vi "SetupInterf.vi"(8 "error in (no error)":errorcluster caption="entrée d'erreur (pas d'erreur)", 9 "Experiment.lvclass":refnum<class "Experiment.lvclass">=refnum, 11 "Interface en entrée":refnum<class "Interface.lvclass"> caption="Interface Class in") -> (0 "error out":errorcluster caption="sortie d'erreur", 3 "Interface en sortie":refnum<class "Interface.lvclass"> caption="DNL_LabVIEW Object out")   [LabVIEW 2019, in "Interface.lvclass"]
uses:
  Interface.lvclass
  Experiment Class/Experiment.lvclass
  DevicesClass/Tools/Tools.lvclass
  CurveSetup.ctl
  SetupInterfStates.ctl
  Interface.lvclass/Interface.ctl
  SetInitPar.ctl
  2DGraphSetup.ctl
  DevicesClass/BaseDevice/BaseDevice.lvclass
panel:
  out "ScanInstrInd":i32[][](array[numeric])
  out "ArrDev":bool[](array[boolean])
  in  "EditArrDev":bool
  out "2D Scan":bool
  in  "2D Plot Act":bool caption="2D Plot"
  out "Fill Line First":bool
  in  "2D Plot":bool
  in  "2D YScanPar":u16(ring) caption="Y Parameter" items=["Selectionner un Paramètre..", "Tools.ScanPar(Arb)"]
  in  "2D XScanPar":u16(ring) caption="X Parameter" items=["Selectionner un Paramètre..", "Tools.Ind Point(Point)", "Tools.ScanPar(Arb)"]
  in  "Data Only":bool
  in  "SaveNamingPar":bool
  out "GraphIndex":i32
  in  "SetGraphConf":bool
  out "Graph Config":i32
  in  "2ndVarParPos":bool=TRUE caption="2nd Scan Parameter Position"
  in  "2ndScanParName":bool=TRUE caption="2nd Scan Parameter Name"
  in  "ParamNaming":bool caption="Use Parameterize Naming"
  in  "YScale":u32(ring) items=["Left 1", "Left 2", "Left 3", "Right 1", "Right 2", "Right 3"]
  in  "X Scale":u32(ring) items=["Bottom", "Top"]
  in  "ScanInstrName":bool=TRUE
  in  "Scan/Log Suffix":bool=TRUE
  in  "MeasUnits":bool=TRUE caption="Measurement Units"
  in  "MeasInstrName":bool=TRUE
  in  "SaveCurvePar":bool
  in  "DisplayName":string
  in  "Visible":bool
  out "CrvParOut":T1[](array[typedef])
  out "NomDon":string[](array[string])=["RTêta;", "X&Y;"]
  out "VarParams":string[][](array[string])
  in  "AutoColor":bool caption="Use Automatic Color"
  out "Graphe XY":cluster{dbl, dbl}[](graph)
  in  "ScanParam":u16(ring) caption="Scan Parameter" items=["Tools.Ind Point(Point)"]
  in  "YScaleName":string
  in  "XScaleName":string
  in  "Graph Window":i32(ring) items=["Graph 0", "No Graph", "New Graph Window "]
  in  "stop":bool
  in  "Curve List":i32(listbox)
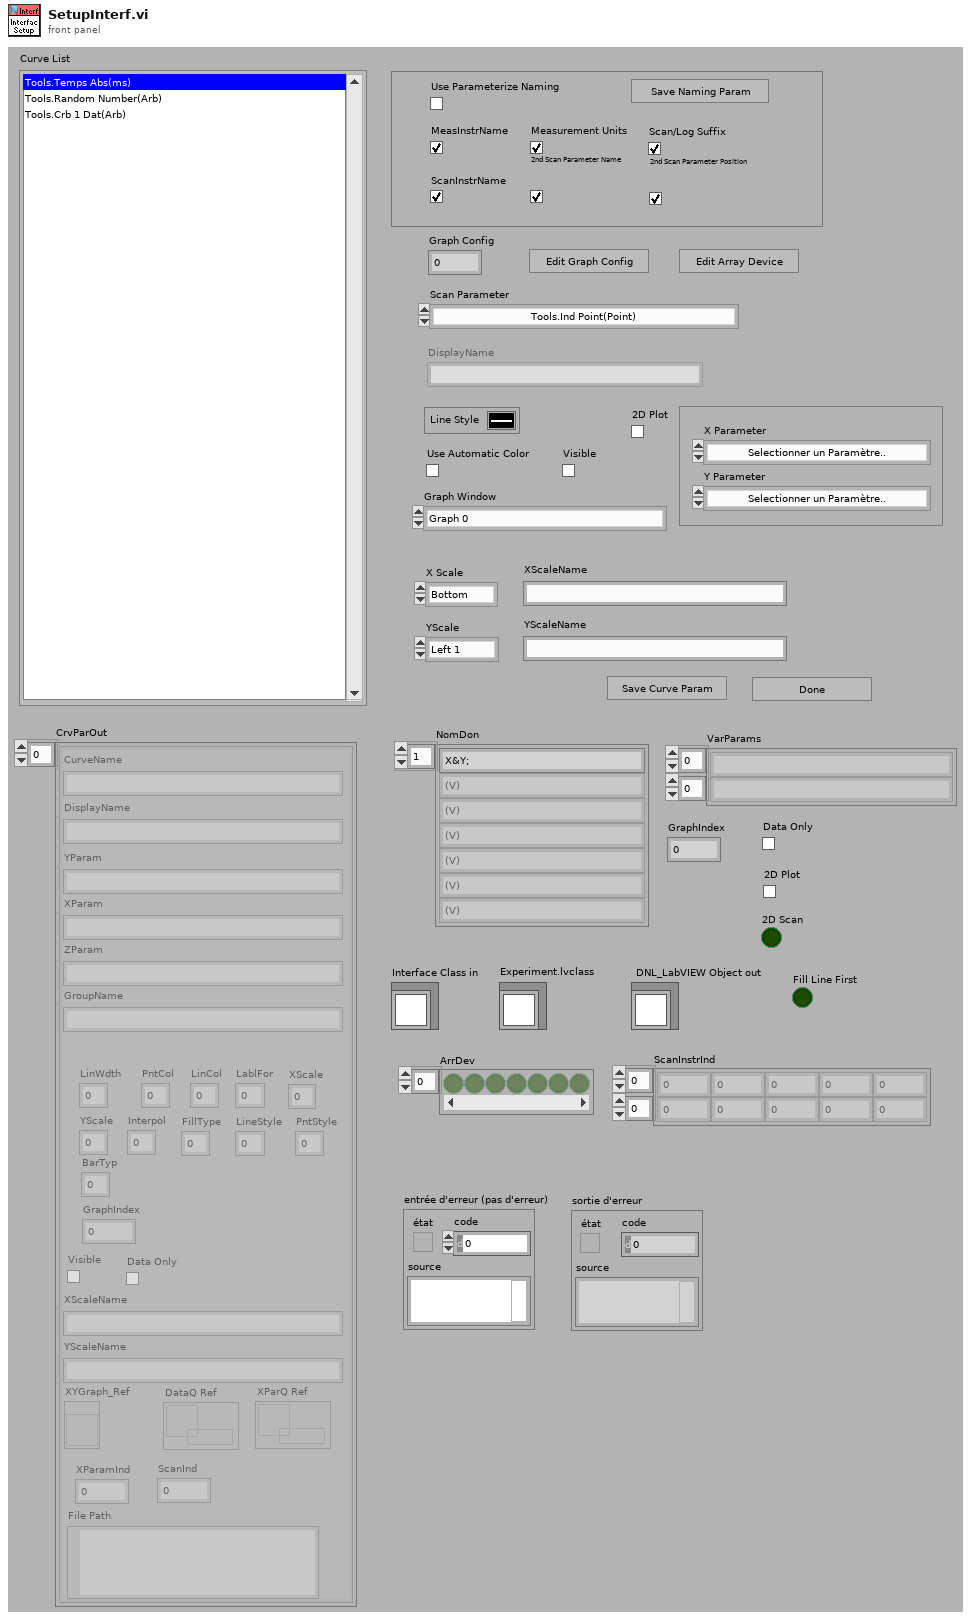
[diagram p1: front panel]
types:
  T1 = typedef "Interface.lvclass/CurveSetup.ctl" = cluster{"CurveName":string, "YParam":string, "XParam":string, "ZParam ":string, "GroupName":string, "LinWdth":u8, "PntCol":u32, "LinCol":u32, "LablFor":u8, "XScale":u32, "YScale":u32, "Interpol":u8, "DisplayName":string, "FillType":i16, "LineStyle":u8, "PntStyle":u8, "BarTyp":u8, "GraphIndex":i32, "Visible":bool, "XScaleName":string, "YScaleName":string, "XYGraph_Ref":refnum<vi>, "Data Only":bool, "DataQ Ref":refnum<queue>, "XParQ Ref":refnum<queue>, "XParamInd":i32, "ScanInd":i32, "File Path":path}
  T2 = typedef "SetInitPar.ctl" = enum16{"All", "AllowSave", "GraphConfig", "ScanFormats", "ScanPref", "LogPref", "BasePath", "Experiment", "SubFolder"}
  T3 = cluster{"MeasInstrNm":bool, "MeasUnits":bool, "ScanSuff":bool, "ScanParNm":bool, "2ndScnParNm":bool, "2ndScnParPos":bool}
  T4 = typedef "SetupInterfStates.ctl" = enum16{"InitProg", "ReadMeasPar", "ReadCurvePar", "ReadGraphPar", "GetScaleName", "ChgScaleName", "ChngGraphConf", "2D Graph", "SaveParams", "SaveParamsDef", "ApplyAll", "ArrDevSetup", "Stop"}
  T5 = enum16{"Enable", "Disable", "DisAndGrayed", "ReinitToDefVal"}
  T6 = enum16{"Enable", "Disable", "DisAndGrayed", "ReinitToDefVal", "EnumElementsArr"}
  T7 = typedef "2DGraphSetup.ctl" = cluster{"ZDataIndex":i32, "XParIndex":i32, "YParIndex":i32, "FillLineFirst":bool, "2DGraphIndex":i32, "XParQ Ref":refnum<queue>, "YParQ Ref":refnum<queue>, "DataQRefs":refnum<queue>[], "CurveName":string, "XparInstrInd":i32, "YparInstrInd":i32, "Active":bool}
  T8 = enum32{"Invalid", "Standard", "Closed", "Hidden", "Minimized", "Maximized"}
  T9 = enum8{"Enabled", "Disabled", "Disabled and Grayed Out"}
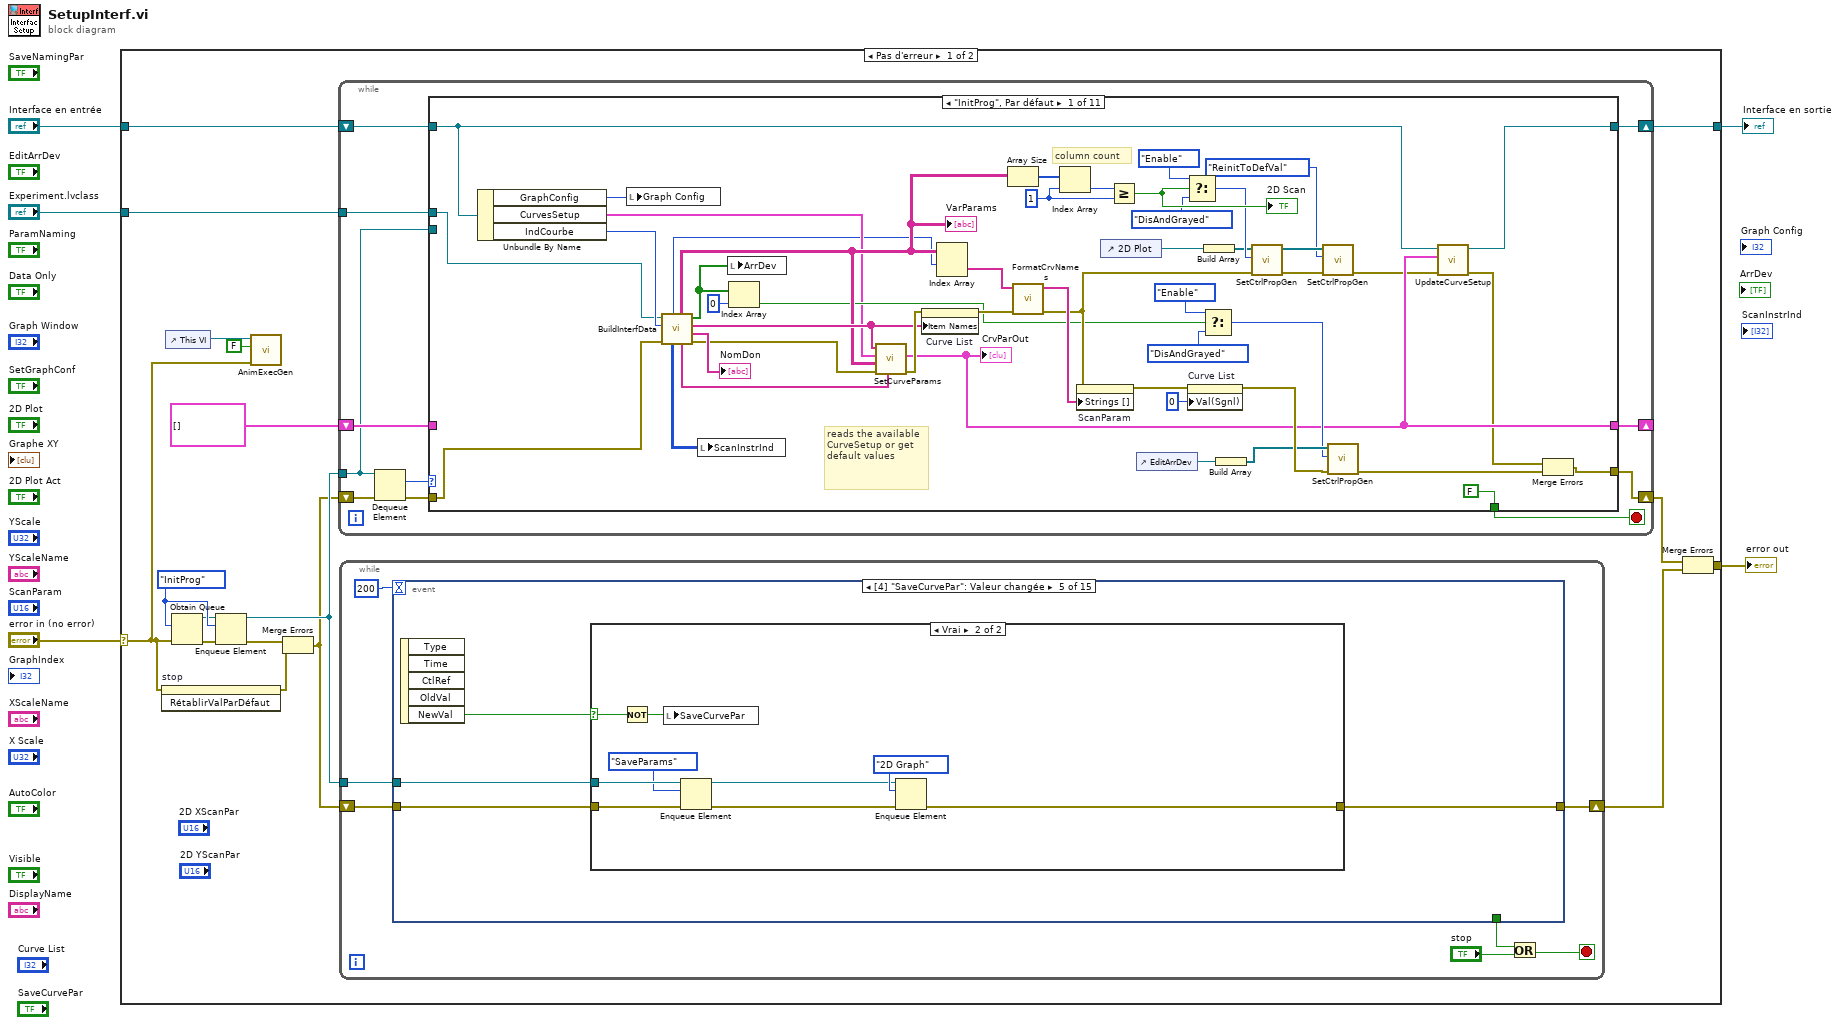
[diagram p0: block diagram]
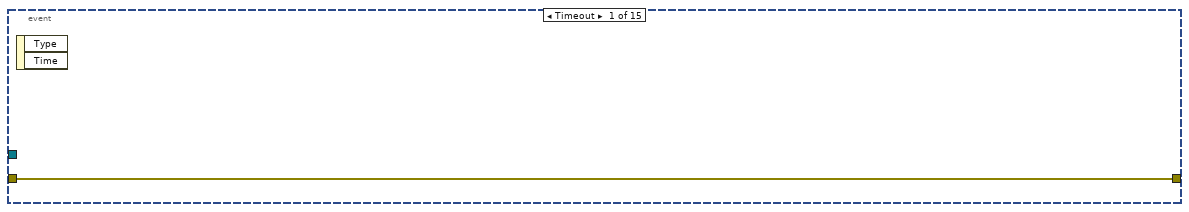
[diagram p2: hidden frame]
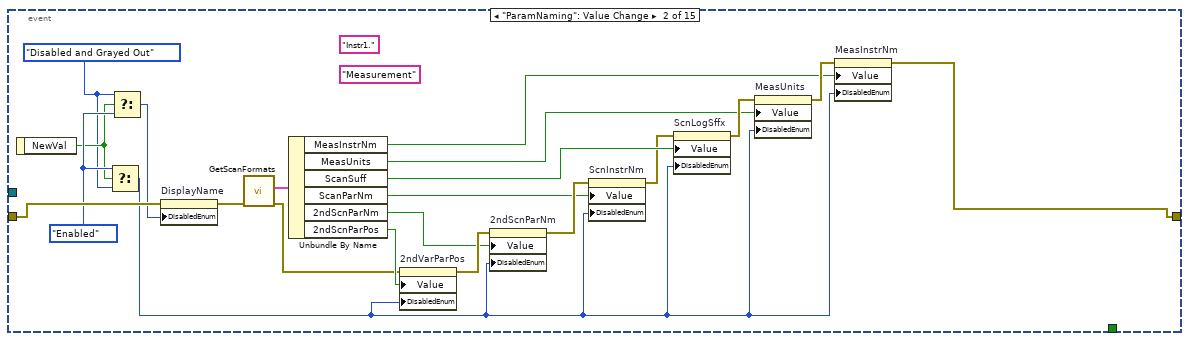
[diagram p3: hidden frame]
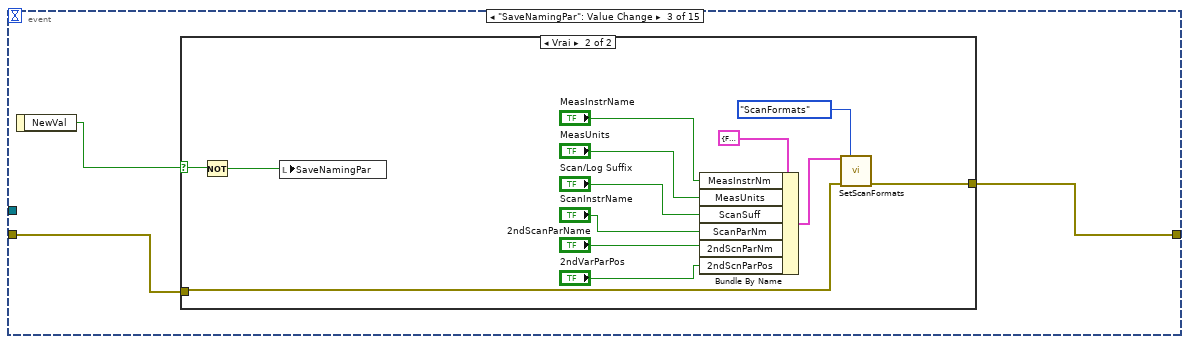
[diagram p4: hidden frame]
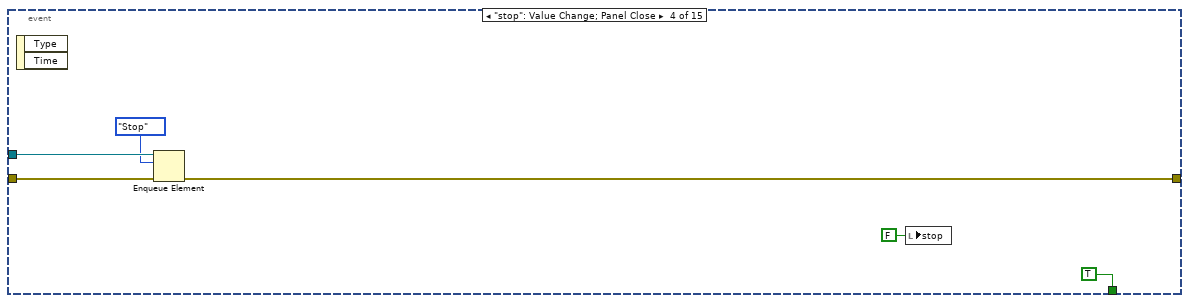
[diagram p6: hidden frame]
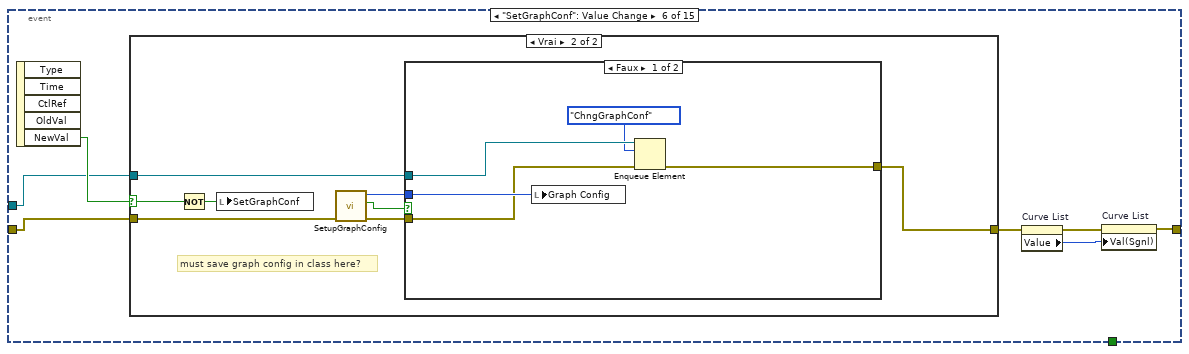
[diagram p8: hidden frame]
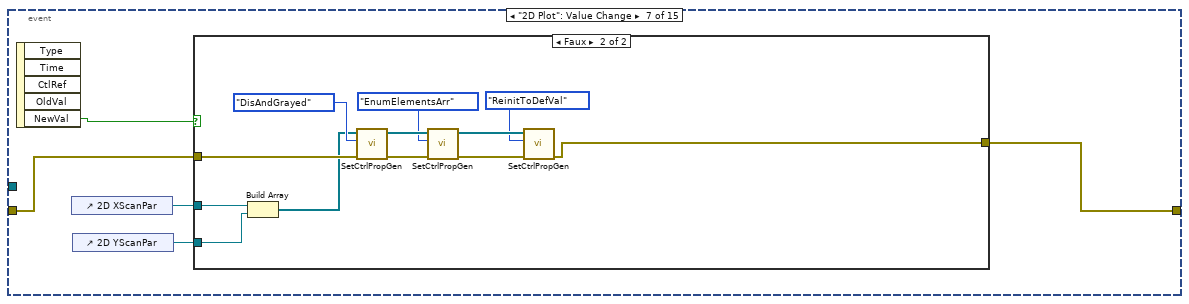
[diagram p11: hidden frame]
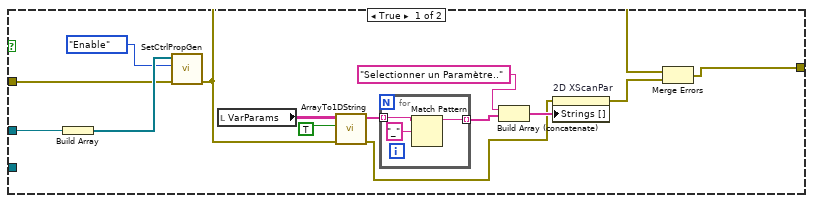
[diagram p12: hidden frame]
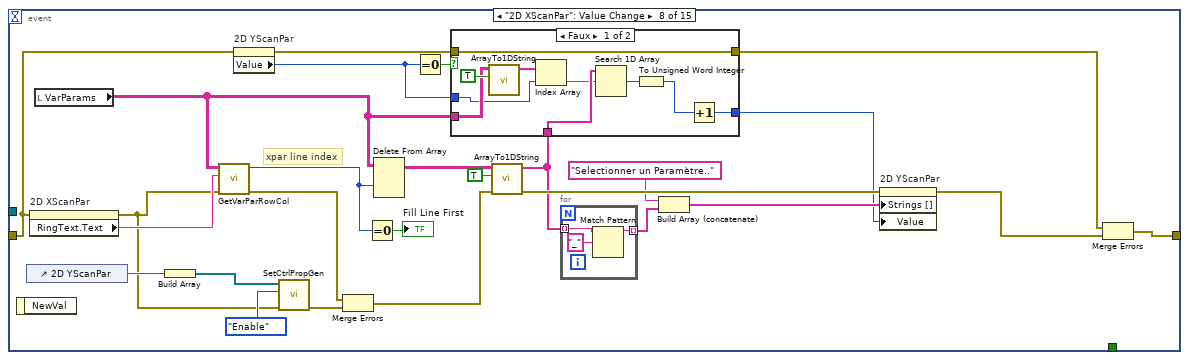
[diagram p13: hidden frame]
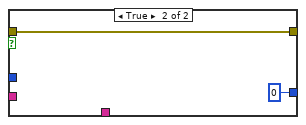
[diagram p14: hidden frame]
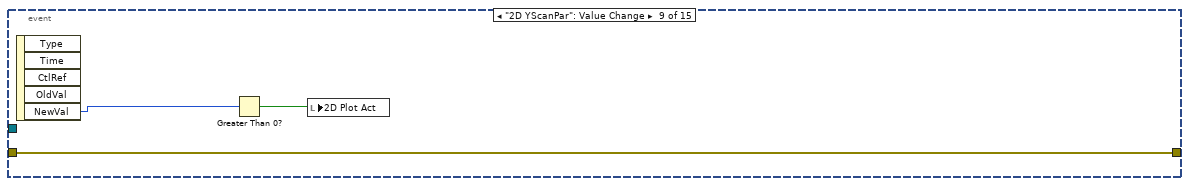
[diagram p15: hidden frame]
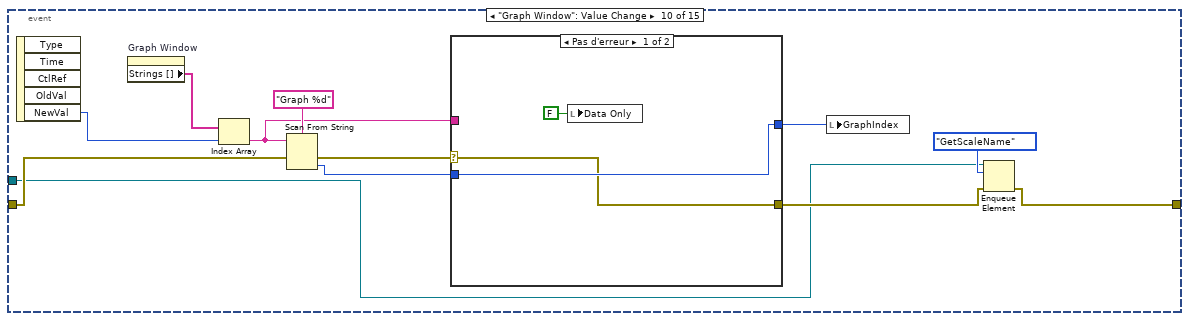
[diagram p16: hidden frame]
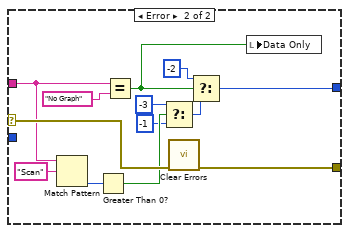
[diagram p17: hidden frame]
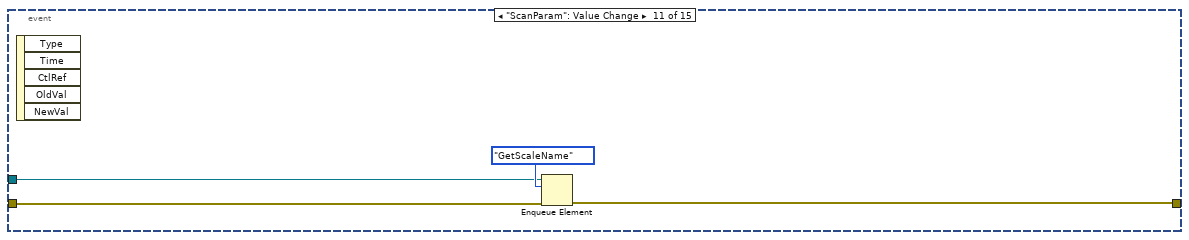
[diagram p18: hidden frame]
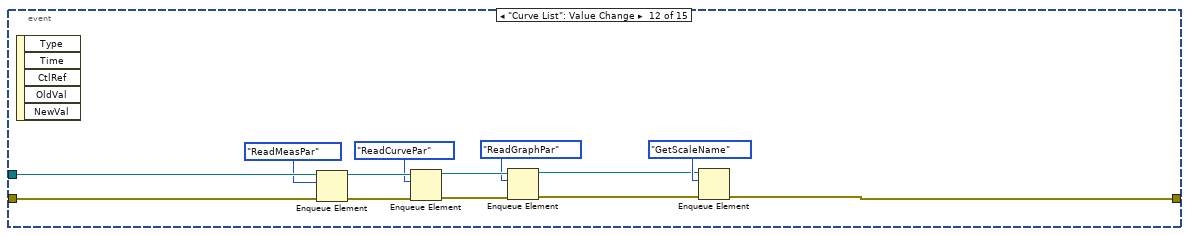
[diagram p19: hidden frame]
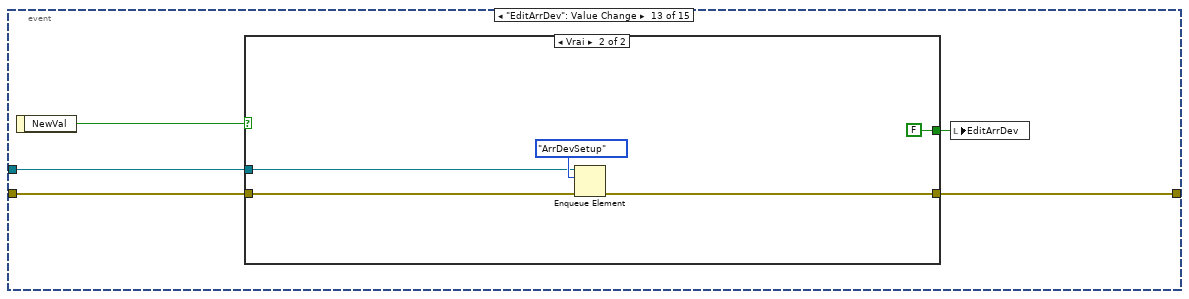
[diagram p20: hidden frame]
diagram:
  n1 = case shown="Pas d'erreur" "error in (no error)" {
    selector: "error in (no error)" -> [w7 w726]
    tunnel: [w11 w726] -> w4
    tunnel: "Interface en entrée" -> [w14 w725]
    tunnel: [w6 w725] -> w2
    tunnel: "Experiment.lvclass" -> [w10 _]
    frame No Error {
      w22 = SetupInterfStates."InitProg" ("Énum")
      n2 = invoke on="stop" class="Bool (strict)" method="RétablirValParDéfaut"(error in=w7) -> (error out=w16:errorcluster)  [unwired: 2 in, 2 out]
      n3 = control-ref of="This VI"() -> (w8:refnum<vi>)
      n4 = Obtain Queue(element data type=w22, error in (no error)=w7) -> (queue out=w21:refnum<queue>, error out=w20:errorcluster)  [unwired: 3 in, 1 out]
      n5 = Enqueue Element(queue=w21, element=w22, error in (no error)=w20) -> (queue out=w19:refnum<queue>, error out=w17:errorcluster)  [unwired: 1 in, 1 out]
      n6 = call <userlib>:"AnimExecGen.vi"("ErrorIn(No Error)"=w7, "Animer l'exécution ?"=FALSE, "ViRef"=w8) -> ()  [unwired: 8 in, 1 out]
      n7 = Merge Errors(w17, w16) -> (w15:errorcluster)
      n8 = while {
        shift-right: [w258] -> w12
        shift-left: w15 -> [w263]
        tunnel: w19 -> [w255]
        shift-right: [w259] -> w6
        shift-left: w14 -> [w262]
        shift-right: [w257] -> _
        shift-left: T1[] [] ("CurveParamsOut") -> [w256]
        tunnel: w10 -> [w254]
        stop <- w260 stop-if-true
        n9 = Dequeue Element(queue=w255, error in (no error)=w263) -> (element=w264:T4, error out=w261:errorcluster)  [unwired: 1 in, 2 out]
        n10 = case shown="\"InitProg\", Par défaut" w264 {
          tunnel: w262 -> [w272 w338 w342 w406 w481 w512 w528 w570 w613 w678 w704]
          tunnel: w261 -> [w267 w332 w365 w425 w492 w519 w530 w567 w631 w672 w693]
          tunnel: [FALSE _ _ _ _ _ _ _ _ TRUE FALSE] -> w260
          tunnel: [w271 w338 w342 w406 w481 w508 w524 w561 w625 w678 w703] -> w259
          tunnel: [w289 w330 w350 w409 w493 w506 w525 w568 w604 w676 w705] -> w258
          tunnel: [w270 w329 w363 w422 w503 w522 w523 w569 w601 w677 w686] -> w257
          tunnel: w256 -> [_ w329 w363 w422 w503 w522 w523 w569 w647 w677 w687]
          tunnel: w255 -> [_ _ _ _ _ _ _ _ _ _ _]
          tunnel: w254 -> [w285 _ _ _ _ _ _ _ _ _ w698]
          frame "InitProg", Default {
            w296 = 1 ("indice")
            # "column count"
            # "reads the available CurveSetup or get default values"
            n11 = Unbundle By Name(w272) -> ("GraphConfig"=w302:i32, "CurvesSetup"=w273:T1[], "IndCourbe"=w301:i64)
            n12 = local write "Graph Config"(w302) -> ()
            n13 = call "BuildInterfData.vi"("error in"=w267, "IndCourbe"=w301, "Experiment.lvclass In"=w285) -> ("error out"=w304:errorcluster, "NomDon"=→"NomDon":string[], "Scan list"=w303:string[], "ArrDev"=w275:bool[], "VarPar list"=w274:string[], "VarParams"=w300:string[][], "ScanInstIndexOut"=w266:i32[][], "firstenableSProw"=w265:i32)  [unwired: 1 in]
            "VarParams" <- w300
            n14 = local write "ScanInstrInd"(w266) -> ()
            n15 = local write "ArrDev"(w275) -> ()
            n16 = Index Array(array=w275, index=0 ("indice")) -> (element=w279:bool)
            n17 = call "SetCurveParams.vi"("VarPar list"=w274, "error in (no error)"=w304, "VarParams"=w300, "CurveSetupsIn"=w273, "CurveNames"=w303) -> ("error out"=w311:errorcluster, "CurveSetupsOut"=w270:T1[])  [unwired: 5 in]
            "CrvParOut" <- w270
            n18 = property on="Curve List" class="LstDér (strict)"(error in=w311, "Item Names"=w303) -> (error out=w305:errorcluster)  [unwired: 1 in, 1 out]
            n19 = Index Array(array=w300, index (row)=w265) -> (element=w307:string[])  [unwired: 1 in]
            n20 = Array Size(array=w300) -> (size(s)=w299:i32[])
            n21 = call "FormatCrvNames.vi"("entrée d'erreur"=w305, "CurveNamesIn"=w307) -> ("sortie d'erreur"=w290:errorcluster, "CurveNames"=w306:string[])  [unwired: 8 in]
            n22 = Index Array(array=w299, index=w296) -> (element=w297:i32)
            n23 = property on="ScanParam" class="MDér (strict)"(error in=w290, "Strings []"=w306) -> (error out=w308:errorcluster)  [unwired: 1 in, 1 out]
            n24 = control-ref of="2D Plot"() -> (w291:refnum<vi>)
            n25 = Greater Or Equal?(x=w297, y=w296) -> (x >= y?=w298:bool)
            "2D Scan" <- w298
            n26 = control-ref of="EditArrDev"() -> (w281:refnum<vi>)
            n27 = Select(t=T5."Enable" ("Énum"), s=w298, f=T5."DisAndGrayed" ("Énum")) -> (s? t:f=w294:T5)
            n28 = property on="Curve List" class="LstDér (strict)"(error in=w308, "Val(Sgnl)"=0 ("Valeur (Signalisation)")) -> (error out=w283:errorcluster)  [unwired: 1 in, 1 out]
            n29 = Select(t=T5."Enable" ("Énum"), s=w279, f=T5."DisAndGrayed" ("Énum")) -> (s? t:f=w276:T5)
            n30 = Build Array(w291) -> (w293:refnum<vi>[])
            n31 = Build Array(w281) -> (w280:refnum<vi>[])
            n32 = call <userlib>:"SetCtrlPropGen.vi"("Error in"=w290, "Énum"=w294, "Controls"=w293) -> ("Error out"=w286:errorcluster, "Controls Out"=w288:refnum<vi>[])  [unwired: 3 in]
            n33 = call <userlib>:"SetCtrlPropGen.vi"("Error in"=w286, "Énum"=T5."ReinitToDefVal", "Controls"=w288) -> ("Error out"=w269:errorcluster)  [unwired: 3 in, 1 out]
            n34 = call <userlib>:"SetCtrlPropGen.vi"("Error in"=w283, "Énum"=w276, "Controls"=w280) -> ("Error out"=w282:errorcluster)  [unwired: 3 in, 1 out]
            n35 = call "UpdateCurveSetup.vi"("ErrorIn(No Error)"=w269, "CurveSetupsIn"=w270, "Interface.lvclass"=w272) -> ("sortie d'erreur"=w268:errorcluster, "Interface.lvclass Out"=w271:refnum<class "Interface.lvclass">)  [unwired: 7 in]
            n36 = Merge Errors(w268, w282) -> (w289:errorcluster)
          }
          frame "ReadMeasPar" {
            n37 = property on="Curve List" class="LstDér (strict)"(error in=w332) -> (error out=w314:errorcluster, "Value"=w316:i32)  [unwired: 1 in, 1 out]
            n38 = local read "ArrDev"() -> (w317:bool[])
            n39 = control-ref of="EditArrDev"() -> (w321:refnum<vi>)
            n40 = Index Array(array=w317, index=w316) -> (element=w315:bool)
            n41 = Build Array(w321) -> (w320:refnum<vi>[])
            n42 = Select(t=T5."Enable" ("Énum"), s=w315, f=T5."DisAndGrayed" ("Énum")) -> (s? t:f=w322:T5)
            n43 = call <userlib>:"SetCtrlPropGen.vi"("Error in"=w314, "Énum"=w322, "Controls"=w320) -> ("Error out"=w313:errorcluster)  [unwired: 3 in, 1 out]
            n44 = Index Array(array=w329, index=w316) -> (element=w331:T1)
            n45 = property on="ScanParam" class="MDér (strict)"(error in=w313) -> (error out=w324:errorcluster, "Strings []"=w333:string[])  [unwired: 1 in, 1 out]
            n46 = Unbundle By Name(w331) -> ("XParam"=w328:string)  [unwired: 1 out]
            n47 = Build Array(w328) -> (w327:string[])
            n48 = call "FormatCrvNames.vi"("entrée d'erreur"=w324, "CurveNamesIn"=w327) -> ("sortie d'erreur"=w323:errorcluster, "CurveNames"=w326:string[])  [unwired: 8 in]
            n49 = Index Array(array=w326) -> (element=w325:string)  [unwired: 1 in]
            n50 = Search 1D Array(1D array=w333, element=w325) -> (index of element=w336:i32)  [unwired: 1 in]
            n51 = Greater Or Equal To 0?(x=w336) -> (x >= 0?=w334:bool)
            n52 = Select(t=w336, s=w334, f=0 ("cas faux")) -> (s? t:f=w337:i32)
            n53 = property on="ScanParam" class="MDér (strict)"(error in=w323, "Value"=w337) -> (error out=w330:errorcluster)  [unwired: 1 in, 1 out]
          }
          frame "ReadCurvePar" {
            n54 = Unbundle By Name(w342) -> ("2DGphParams"=w343:T7[])
            n55 = property on="Curve List" class="LstDér (strict)"(error in=w365) -> (error out=w353:errorcluster, "Item Names"=w347:string[], "Value"=w345:i32)  [unwired: 1 in, 1 out]
            n56 = Index Array(array=w347, index=w345) -> (element=w346:string)
            n57 = Index Array(array=w363, index=w345) -> (element=w366:T1)
            n58 = for {
              tunnel: w343 -> [w380] mode=indexing
              tunnel: w346 -> [w378]
              tunnel: [w377] -> w344
              tunnel: [w376] -> w341
              tunnel: [w375] -> w340
              i -> [w377]
              stop <- w376 stop-if-true
              n59 = Unbundle By Name(w380) -> ("Active"=w375:bool, "CurveName"=w379:string)
              n60 = Equal?(x=w379, y=w378) -> (x = y?=w376:bool)
            }
            n61 = Unbundle By Name(w366) -> ("PntCol"=w362:u32, "LinCol"=w361:u32)
            n62 = And(x=w340, y=w341) -> (x .and. y?=w339:bool)
            n63 = Unbundle By Name(w366) -> ("LinWdth"=w374:u8, "LablFor"=w368:u8)
            n64 = Unbundle By Name(w366) -> ("Interpol"=w369:u8, "FillType"=w370:i16, "LineStyle"=w371:u8, "PntStyle"=w372:u8, "BarTyp"=w373:u8)
            n65 = call "GetPlotColors.vi"("Color2In"=w361, "Color1In"=w362, "ColorIndex"=0) -> ("Color2Out"=w357:u32, "Color1Out"=w358:u32, "AutoColor"=w359:bool)  [unwired: 5 in, 1 out]
            n66 = local write "AutoColor"(w359) -> ()
            n67 = Index Array(array=w343, index=w344) -> (element=w348:T7)
            n68 = property on="Graphe XY" class="GraphXY (strict)"(error in=w353, "Active Plot"=u32 0 ("Tracé actif"), "Plot.Fill/Pt. Color"=w358, "Plot.Plot Color"=w357, "Plot.Line Width"=w374, "Plot.Label Style"=w368, "Plot.Plot Interpolation"=w369, "Plot.Fill To"=w370, "Plot.Line Style"=w371, "Plot.Point Style"=w372, "Plot.Bar Plot Style"=w373) -> (error out=w364:errorcluster)  [unwired: 1 in, 1 out]
            n69 = Unbundle By Name(w348) -> ("ZDataIndex"=w354:i32, "XParIndex"=w352:i32, "YParIndex"=w351:i32)
            n70 = call <vilib>:"General Error Handler.vi"("error in (no error)"=w364) -> ("error out"=w356:errorcluster)  [unwired: 10 in, 4 out]
            n71 = case shown="Vrai" w339 {
              tunnel: w354 -> [_ _]
              tunnel: w353 -> [w382 w389]
              tunnel: w352 -> [_ w392]
              tunnel: w351 -> [_ w385]
              tunnel: [w381 w387] -> w349
              frame False {
                n72 = property on="2D Plot" class="Bool (strict)"(error in=w382, "Val(Sgnl)"=FALSE ("Valeur (Signalisation)")) -> (error out=w381:errorcluster)  [unwired: 1 in, 1 out]
              }
              frame True {
                n73 = property on="2D Plot" class="Bool (strict)"(error in=w389, "Val(Sgnl)"=TRUE ("Valeur (Signalisation)")) -> (error out=w393:errorcluster)  [unwired: 1 in, 1 out]
                n74 = Increment(x=w392) -> (x+1=w391:i32)
                n75 = To Unsigned Word Integer(number=w391) -> (unsigned 16bit integer=w390:u16)
                n76 = property on="2D XScanPar" class="MDér (strict)"(error in=w393, "Val(Sgnl)"=w390) -> (error out=w388:errorcluster)  [unwired: 1 in, 1 out]
                n77 = To Unsigned Word Integer(number=w385) -> (unsigned 16bit integer=w384:u16)
                n78 = property on="2D YScanPar" class="MDér (strict)"(error in=w388, "Value"=w384) -> (error out=w387:errorcluster)  [unwired: 1 in, 1 out]
              }
            }
            n79 = local write "2D Plot Act"(w339) -> ()
            n80 = call <vilib>:"Clear Errors.vi"("error in (no error)"=w356) -> ("error out"=w355:errorcluster)  [unwired: 5 in, 1 out]
            n81 = Merge Errors(w349, w355) -> (w350:errorcluster)
          }
          frame "ReadGraphPar" {
            n82 = local read "Graph Config"() -> (w399:i32)
            n83 = property on="Curve List" class="LstDér (strict)"(error in=w425) -> (error out=w416:errorcluster, "Value"=w405:i32)  [unwired: 1 in, 1 out]
            n84 = Index Array(array=w422, index=w405) -> (element=w423:T1)
            n85 = local read "2D Scan"() -> (w395:bool)
            n86 = Unbundle By Name(w423) -> ("GraphIndex"=w417:i32)
            n87 = call "GraphConfCount.vi"("Configuration"=w399) -> ("GraphCount"=w398:i32)  [unwired: 9 in, 1 out]
            n88 = To Long Integer(number=w398) -> (32bit integer=w418:i32)
            n89 = Greater Or Equal To 0?(x=w417) -> (x >= 0?=w419:bool)
            n90 = Select(t=string[] ["No Graph", "New Graph Window For Each Curve", "New Graph Window For Each Scan"], s=w395, f=string[] ["No Graph", "New Graph Window "]) -> (s? t:f=w397:string[])
            n91 = case shown="Vrai" w419 {
              tunnel: w418 -> [w428 w455]
              tunnel: w417 -> [w426 w457]
              tunnel: [w433 w460] -> w415
              tunnel: w416 -> [w432 w459]
              tunnel: [w430 w458] -> w414
              tunnel: w397 -> [w429 w454]
              tunnel: [w431 w456] -> w413
              tunnel: [w427 w453] -> w412
              frame False {
                # "either new window (-1,-3) or no window(-2)"
                n92 = Equal?(x=w426, y=-2) -> (x = y?=w434:bool)
                n93 = case shown="Faux" w434 {
                  tunnel: [w446 w452] -> w433
                  tunnel: w432 -> [w446 w452]
                  tunnel: w428 -> [w445 w451]
                  tunnel: [w448 w451] -> w431
                  tunnel: [w447 w450] -> w430
                  tunnel: w429 -> [w447 w450]
                  tunnel: [w438 -2] -> w427
                  tunnel: w426 -> [w444 _]
                  frame False {
                    n94 = Equal?(x=w444, y=-1) -> (x = y?=w439:bool)
                    n95 = Select(t=1 ("y"), s=w439, f=2 ("y")) -> (s? t:f=w440:i32)
                    n96 = Select(t=-1, s=w439, f=-3) -> (s? t:f=w438:i32)
                    n97 = Add(x=w445, y=w440) -> (x+y=w448:i32)
                  }
                  frame True {
                    # "No graph"
                  }
                }
              }
              frame True {
                # "either valid or invalid (absent) graph window"
                n98 = Less Or Equal?(x=w455, y=w457) -> (x <= y?=w461:bool)
                n99 = case shown="Vrai" w461 {
                  tunnel: w459 -> [w464 w473]
                  tunnel: [w464 w472] -> w460
                  tunnel: [w463 w470] -> w458
                  tunnel: w454 -> [w463 w469]
                  tunnel: w457 -> [w462 w465]
                  tunnel: [w462 w466] -> w456
                  tunnel: w455 -> [_ w468]
                  tunnel: [w462 w465] -> w453
                  frame False {
                  }
                  frame True {
                    n100 = Add(x=w468, y=2) -> (x+y=w466:i32)
                    n101 = Format Into String(format string="Graph %d (unavailable)" ("chaîne de format"), error in=w473, w465) -> (resulting string=w471:string, error out=w472:errorcluster)  [unwired: 1 in]
                    n102 = Build Array (concatenate)(w469, w471) -> (w470:string[])
                  }
                }
              }
            }
            n103 = for {
              N: w418 -> [_]
              tunnel: [w475] -> w421 mode=indexing
              i -> [w477]
              n104 = Format Into String(format string="Graph %d" ("chaîne de format"), w477) -> (resulting string=w475:string)  [unwired: 2 in, 1 out]
            }
            n105 = local write "GraphIndex"(w412) -> ()
            n106 = Unbundle By Name(w423) -> ("Data Only"=w408:bool, "DisplayName"=w411:string, "Visible"=w424:bool, "XScale"=w402:u32, "YScale"=w401:u32)
            n107 = Build Array (concatenate)(w421, w414) -> (w420:string[])
            n108 = property on="Graph Window" class="MDér (strict)"(error in=w415, "Strings []"=w420, "Value"=w413) -> (error out=w400:errorcluster)  [unwired: 1 in, 1 out]
            n109 = Empty String/Path?(string/path=w411) -> (empty?=w410:bool)
            n110 = local write "Data Only"(w408) -> ()
            n111 = local write "DisplayName"(w411) -> ()
            n112 = local write "Visible"(w424) -> ()
            n113 = property on="X Scale" class="MDér (strict)"(error in=w400, "Value"=w402) -> (error out=w404:errorcluster)  [unwired: 1 in, 1 out]
            n114 = property on="YScale" class="MDér (strict)"(error in=w400, "Value"=w401) -> (error out=w403:errorcluster)  [unwired: 1 in, 1 out]
            n115 = Merge Errors(w404, w403) -> (w407:errorcluster)
            n116 = property on="ParamNaming" class="Bool (strict)"(error in=w407, "Val(Sgnl)"=w410) -> (error out=w409:errorcluster)  [unwired: 1 in, 1 out]
          }
          frame "GetScaleName" {
            # "if you don't \"save param\"\ngraph stays with no scale"
            # "The first data element gives is names to the y scale #0\nThe first varpar gives is name to the x scale #0\nOther scale number get their names attributed at selection"
            n117 = property on="GraphIndex" class="NumNb (strict)"(error in=w492) -> ("Value"=w487:i32)  [unwired: 1 in, 2 out]
            n118 = property on="Curve List" class="LstDér (strict)"(error in=w492) -> (error out=w479:errorcluster, "Value"=w504:i32)  [unwired: 1 in, 1 out]
            n119 = Index Array(array=w503, index=w504) -> (element=w499:T1)
            n120 = property on="ScanParam" class="MDér (strict)"(error in=w479) -> (error out=w478:errorcluster, "RingText.Text"=w480:string)  [unwired: 1 in, 1 out]
            n121 = Unbundle By Name(w499) -> ("CurveName"=w496:string)
            n122 = property on="X Scale" class="MDér (strict)"(error in=w479) -> (error out=w495:errorcluster, "Value"=w490:u32)  [unwired: 1 in, 1 out]
            n123 = property on="YScale" class="MDér (strict)"(error in=w479) -> (error out=w494:errorcluster, "Value"=w485:u32)  [unwired: 1 in, 1 out]
            n124 = Unbundle By Name(w481) -> ("XScalesNames"=w491:string[][], "YScalesNames"=w486:string[][])
            n125 = Merge Errors(w478, w495, w494) -> (w493:errorcluster)
            n126 = Index Array(array=w486, index (row)=w487, index (col)=w485) -> (element=w484:string)
            n127 = Index Array(array=w491, index (row)=w487, index (col)=w490) -> (element=w501:string)
            n128 = Match Pattern(string=w496, regular expression="_" ("expression régulière")) -> (before substring=w497:string)  [unwired: 1 in, 3 out]
            n129 = Match Pattern(string=w480, regular expression="_" ("expression régulière")) -> (before substring=w498:string)  [unwired: 1 in, 3 out]
            n130 = Empty String/Path?(string/path=w501) -> (empty?=w483:bool)
            n131 = Empty String/Path?(string/path=w484) -> (empty?=w482:bool)
            n132 = Select(t=w497, s=w482, f=w484) -> (s? t:f=w488:string)
            n133 = Select(t=w498, s=w483, f=w501) -> (s? t:f=w489:string)
            n134 = local write "YScaleName"(w488) -> ()
            n135 = local write "XScaleName"(w489) -> ()
          }
          frame "ChgScaleName" {
            n136 = Unbundle By Name(w512) -> ("XScalesNames"=w516:string[][], "YScalesNames"=w515:string[][])
            n137 = property on="X Scale" class="MDér (strict)"(error in=w519) -> (error out=w511:errorcluster, "Value"=w518:u32)  [unwired: 1 in, 1 out]
            n138 = property on="YScale" class="MDér (strict)"(error in=w519) -> (error out=w510:errorcluster, "Value"=w517:u32)  [unwired: 1 in, 1 out]
            n139 = Merge Errors(w511, w510) -> (w505:errorcluster)
            n140 = local read "GraphIndex"() -> (w507:i32)
            n141 = local read "YScaleName"() -> (w521:string)
            n142 = local read "XScaleName"() -> (w520:string)
            n143 = Replace Array Subset(array=w516, new element=w520, index (row)=w507, index (col)=w518) -> (w513:string[][])
            n144 = Replace Array Subset(array=w515, new element=w521, index (row)=w507, index (col)=w517) -> (w514:string[][])
            n145 = Bundle By Name(cluster=w512, "XScalesNames"=w513, "YScalesNames"=w514) -> (w509:refnum<class "Interface.lvclass">)
            n146 = call "SetGrphScale.vi"("error in (no error)"=w505, "GraphIndex"=w507, "Interface en entrée"=w509) -> ("error out"=w506:errorcluster, "Interface en sortie"=w508:refnum<class "Interface.lvclass">)  [unwired: 7 in]
          }
          frame "ChngGraphConf" {
            n147 = local read "Graph Config"() -> (w527:i32)
            n148 = call "SetScanFormats.vi"("Énum"=SetInitPar."GraphConfig", "ErrorIn(No Error)"=w530, "GraphConfig"=w527) -> ("sortie d'erreur"=w526:errorcluster)  [unwired: 12 in]
            n149 = call "ChangeGraphConfig.vi"("error in (no error)"=w526, "NewGraphConfig"=w527, "Interface en entrée"=w528) -> ("error out"=w525:errorcluster, "Interface en sortie"=w524:refnum<class "Interface.lvclass">)  [unwired: 7 in]
          }
          frame "2D Graph" {
            n150 = Unbundle By Name(w570) -> ("2DGphParams"=w563:T7[])
            n151 = property on="Curve List" class="LstDér (strict)"(error in=w567) -> (error out=w566:errorcluster, "Value"=w565:i32, "Item Names"=w564:string[])  [unwired: 1 in, 1 out]
            n152 = local read "VarParams"() -> (w538:string[][])
            n153 = call <userlib>:"ArrayTo1DString.vi"("ErrorIn(No Error)"=w566, "DelArrEnd(F)"=TRUE ("DelArrEnd"), "tableau"=w538) -> ("sortie d'erreur"=w550:errorcluster, "Array Out"=w555:string[])  [unwired: 6 in, 1 out]
            n154 = property on="2D XScanPar" class="MDér (strict)"(error in=w566) -> (error out=w540:errorcluster, "Value"=w559:u16, "RingText.Text"=w539:string)  [unwired: 1 in, 1 out]
            n155 = property on="2D YScanPar" class="MDér (strict)"(error in=w566) -> (error out=w549:errorcluster, "RingText.Text"=w544:string)  [unwired: 1 in, 1 out]
            n156 = for {
              tunnel: w555 -> [w600] mode=indexing
              tunnel: [w599] -> w554 mode=indexing
              n157 = Match Pattern(string=w600, regular expression="_" ("expression régulière")) -> (before substring=w599:string)  [unwired: 1 in, 3 out]
            }
            n158 = call "GetVarParRowCol.vi"("ErrorIn(No Error)"=w566, "VarPar"=w539, "VarParams"=w538) -> ("sortie d'erreur"=w537:errorcluster, "Col"=w535:i32, "Line"=w534:i32)  [unwired: 6 in]
            n159 = call "GetVarParRowCol.vi"("ErrorIn(No Error)"=w566, "VarPar"=w544, "VarParams"=w538) -> ("sortie d'erreur"=w536:errorcluster, "Col"=w532:i32, "Line"=w533:i32)  [unwired: 6 in]
            n160 = Search 1D Array(1D array=w554, element=w544) -> (index of element=w553:i32)  [unwired: 1 in]
            n161 = Merge Errors(w550, w549, w540) -> (w548:errorcluster)
            n162 = Index Array(array=w564, index=w565) -> (element=w547:string)
            n163 = local read "ScanInstrInd"() -> (w542:i32[][])
            n164 = Merge Errors(w548, w537, w536) -> (w568:errorcluster)
            n165 = Index Array(array=w542, index (row)=w534, index (col)=w535) -> (element=w541:i32)
            n166 = Index Array(array=w542, index (row)=w533, index (col)=w532) -> (element=w543:i32)
            n167 = local read "2D Plot"() -> (w531:bool)
            n168 = local read "Fill Line First"() -> (w557:bool)
            n169 = for {
              tunnel: w563 -> [w597] mode=indexing
              tunnel: w547 -> [w595]
              tunnel: [w594] -> w545
              tunnel: [w593] -> w546
              i -> [w594]
              stop <- w593 stop-if-true
              n170 = Unbundle By Name(w597) -> ("CurveName"=w596:string)
              n171 = Equal?(x=w596, y=w595) -> (x = y?=w593:bool)
            }
            n172 = Decrement(x=w559) -> (x-1=w558:u16)
            n173 = To Long Integer(number=w558) -> (32bit integer=w552:i32)
            n174 = Bundle By Name(cluster=T7 {"ZDataIndex"=0, "XParIndex"=0, "YParIndex"=0, "FillLineFirst"=FALSE, "2DGraphIndex"=0, "XParQ Ref"=refnum, "YParQ Ref"=refnum, "DataQRefs"=[], "CurveName"="", "XparInstrInd"=-1, "YparInstrInd"=-1, "Active"=FALSE} ("2DGphParam"), "CurveName"=w547, "ZDataIndex"=w565, "XParIndex"=w552, "YParIndex"=w553, "FillLineFirst"=w557, "XparInstrInd"=w541, "YparInstrInd"=w543, "Active"=w531) -> (w551:T7)
            n175 = case shown="Vrai" w531 {
              tunnel: w563 -> [w575 w587]
              tunnel: [w574 w586] -> w562
              tunnel: w551 -> [w573 w585]
              tunnel: w546 -> [w572 w584]
              tunnel: w545 -> [w571 w583]
              frame True {
                n176 = case shown="Vrai" w572 {
                  tunnel: w573 -> [w577 w582]
                  tunnel: [w576 w581] -> w574
                  tunnel: w575 -> [w578 w580]
                  tunnel: w571 -> [_ w579]
                  frame False {
                    n177 = Build Array (concatenate)(w578, w577) -> (w576:T7[])
                  }
                  frame True {
                    n178 = Replace Array Subset(array=w580, new element=w582, index=w579) -> (w581:T7[])
                  }
                }
              }
              frame False {
                n179 = case shown="Faux" w584 {
                  tunnel: w585 -> [_ w592]
                  tunnel: [w588 w591] -> w586
                  tunnel: w587 -> [w588 w590]
                  tunnel: w583 -> [_ w589]
                  frame False {
                  }
                  frame True {
                    n180 = Replace Array Subset(array=w590, new element=w592, index=w589) -> (w591:T7[])
                  }
                }
              }
            }
            n181 = Bundle By Name(cluster=w570, "2DGphParams"=w562) -> (w561:refnum<class "Interface.lvclass">)
          }
          frame "SaveParams" {
            n182 = property on="Curve List" class="LstDér (strict)"(error in=w631) -> (error out=w607:errorcluster, "Value"=w646:i32)  [unwired: 1 in, 1 out]
            n183 = local read "GraphIndex"() -> (w609:i32)
            n184 = Unbundle By Name(w613) -> ("XScalesNames"=w619:string[][], "YScalesNames"=w618:string[][])
            n185 = Index Array(array=w647, index=w646) -> (element=w655:T1)
            n186 = local read "YScaleName"() -> (w620:string)
            n187 = property on="X Scale" class="MDér (strict)"(error in=w607) -> (error out=w630:errorcluster, "Value"=w617:u32)  [unwired: 1 in, 1 out]
            n188 = local read "XScaleName"() -> (w621:string)
            n189 = property on="YScale" class="MDér (strict)"(error in=w630) -> (error out=w611:errorcluster, "Value"=w616:u32)  [unwired: 1 in, 1 out]
            n190 = Replace Array Subset(array=w618, new element=w620, index (row)=w609, index (col)=w616) -> (w614:string[][])
            n191 = Replace Array Subset(array=w619, new element=w621, index (row)=w609, index (col)=w617) -> (w615:string[][])
            n192 = Bundle By Name(cluster=w655, "XScale"=w617, "YScale"=w616, "GraphIndex"=w609) -> (w654:T1)
            n193 = Merge Errors(w611) -> (w606:errorcluster)
            n194 = Bundle By Name(cluster=w613, "XScalesNames"=w615, "YScalesNames"=w614) -> (w612:refnum<class "Interface.lvclass">)
            n195 = property on="Graphe XY" class="GraphXY (strict)"(error in=w606, "Active Plot"=u32 0 ("Tracé actif")) -> (error out=w642:errorcluster, "Plot.Fill/Pt. Color"=w652:u32, "Plot.Plot Color"=w651:u32, "Plot.Line Width"=w662:u8, "Plot.Label Style"=w661:u8, "Plot.Plot Interpolation"=w660:u8, "Plot.Fill To"=w659:i16, "Plot.Line Style"=w658:u8, "Plot.Point Style"=w657:u8, "Plot.Bar Plot Style"=w656:u8)  [unwired: 1 in, 1 out]
            n196 = local read "AutoColor"() -> (w653:bool)
            n197 = call "SetGrphScale.vi"("error in (no error)"=w606, "GraphIndex"=w609, "Interface en entrée"=w612) -> ("error out"=w610:errorcluster, "Interface en sortie"=w602:refnum<class "Interface.lvclass">)  [unwired: 7 in]
            n198 = local read "ParamNaming"() -> (w626:bool)
            n199 = case shown="Vrai" w653 {
              tunnel: w654 -> [w669 w671]
              tunnel: w652 -> [w668 _]
              tunnel: w651 -> [w665 _]
              tunnel: [w667 w671] -> w637
              frame False {
                n200 = To Long Integer(number=w668) -> (32bit integer=w666:i32)
                n201 = To Long Integer(number=w665) -> (32bit integer=w664:i32)
                n202 = Bundle By Name(cluster=w669, "PntCol"=w666, "LinCol"=w664) -> (w667:T1)
              }
              frame True {
                w670 = -1 ("PntCol")
                n203 = Bundle By Name(cluster=w671, "PntCol"=w670, "LinCol"=w670) -> ()  [unwired: 1 out]
              }
            }
            n204 = local read "DisplayName"() -> (w629:string)
            n205 = Bundle By Name(cluster=w637, "LinWdth"=w662, "LablFor"=w661, "Interpol"=w660, "FillType"=w659, "LineStyle"=w658, "PntStyle"=w657, "BarTyp"=w656) -> (w644:T1)
            n206 = local read "VarParams"() -> (w635:string[][])
            n207 = Select(t="" ("cas vrai"), s=w626, f=w629) -> (s? t:f=w627:string)
            n208 = property on="Curve List" class="LstDér (strict)"(error in=w642) -> (error out=w624:errorcluster, "Item Names"=w641:string[], "Value"=w640:i32)  [unwired: 1 in, 1 out]
            n209 = property on="ScanParam" class="MDér (strict)"(error in=w642) -> (error out=w638:errorcluster, "Value"=w633:u16)  [unwired: 1 in, 1 out]
            n210 = local read "Visible"() -> (w650:bool)
            n211 = local read "XScaleName"() -> (w649:string)
            n212 = local read "YScaleName"() -> (w648:string)
            n213 = local read "Data Only"() -> (w622:bool)
            n214 = Index Array(array=w635, index (row)=0 ("indice (ligne)")) -> (element=w636:string[])  [unwired: 1 in]
            n215 = To Long Integer(number=w633) -> (32bit integer=w608:i32)
            n216 = Index Array(array=w641, index=w640) -> (element=w639:string)
            n217 = Index Array(array=w636, index=w608) -> (element=w632:string)
            n218 = Bundle By Name(cluster=w644, "CurveName"=w639, "XParam"=w632, "XParamInd"=w608) -> (w643:T1)
            n219 = Bundle By Name(cluster=w643, "DisplayName"=w627, "Visible"=w650, "XScaleName"=w649, "YScaleName"=w648, "Data Only"=w622) -> (w645:T1)
            n220 = local read "Graph Config"() -> (w623:i32)
            n221 = Replace Array Subset(array=w647, new element=w645, index=w646) -> (w601:T1[])
            n222 = Merge Errors(w624, w638, w610) -> (w605:errorcluster)
            n223 = call "UpdateCurveSetup.vi"("ErrorIn(No Error)"=w605, "CurveSetupsIn"=w601, "Interface.lvclass"=w602) -> ("sortie d'erreur"=w604:errorcluster, "Interface.lvclass Out"=w603:refnum<class "Interface.lvclass">)  [unwired: 7 in]
            n224 = Bundle By Name(cluster=w603, "GraphConfig"=w623) -> (w625:refnum<class "Interface.lvclass">)
          }
          frame "Stop" {
            n225 = control-ref of="ce VI"() -> (w675:refnum<vi>)
            n226 = property class="VI"(reference=w675, error in=w672) -> (error out=w673:errorcluster, "FP.State"=w674:T8)  [unwired: 1 out]
            n227 = case shown="\"Standard\", Par défaut" w674 {
              tunnel: [w680 w683] -> w676
              tunnel: w675 -> [_ w682]
              tunnel: w673 -> [w680 w681]
              frame "Closed" {
              }
              frame "Standard", Default {
                n228 = invoke class="VI" method="FA.Fermer"(reference=w682, error in=w681) -> (error out=w683:errorcluster)  [unwired: 1 in, 2 out]
              }
            }
          }
          frame "ArrDevSetup" {
            n229 = property on="Curve List" class="LstDér (strict)"(error in=w693) -> (error out=w685:errorcluster, "Value"=w702:i32, "Item Names"=w701:string[])  [unwired: 1 in, 1 out]
            n230 = property class="Experiment.lvclass"(reference=w698, error in=w685) -> ("Accessor:LoadedInst"=w697:refnum<class "BaseDevice.lvclass">[])  [unwired: 2 out]
            n231 = Index Array(array=w701, index=w702) -> (element=w700:string)
            n232 = Match Pattern(string=w700, regular expression="\\." ("expression régulière")) -> (before substring=w696:string)  [unwired: 1 in, 3 out]
            n233 = for {
              tunnel: w697 -> [w724] mode=indexing
              tunnel: w696 -> [w722]
              tunnel: [w721] -> w695
              tunnel: [w720] -> w689
              shift-right: [w719] -> w694
              shift-left: _ -> [_]
              tunnel: [w718] -> w691
              i -> [w718]
              stop <- w720 stop-if-true
              n234 = property class="BaseDevice.lvclass"(reference=w724) -> (reference out=w721:refnum<class "BaseDevice.lvclass">, error out=w719:errorcluster, "Accessor:InstrumentName"=w723:string)  [unwired: 1 in]
              n235 = Equal?(x=w723, y=w722) -> (x = y?=w720:bool)
            }
            n236 = Not(x=w689) -> (.not. x?=w684:bool)
            n237 = property class="BaseDevice.lvclass"(reference=w695, error in=w694) -> ("Accessor:SubVarParNm X"=w692:string[])  [unwired: 2 out]
            n238 = Empty Array?(array=w692) -> (empty?=w690:bool)
            n239 = Or(x=w690, y=w684) -> (x .or. y?=w688:bool)
            n240 = case shown="Faux" w688 {
              tunnel: [w713 w716] -> w705
              tunnel: w704 -> [w712 w717]
              tunnel: [w707 w717] -> w703
              tunnel: w698 -> [w711 _]
              tunnel: w693 -> [w710 w716]
              tunnel: w691 -> [w709 _]
              tunnel: w687 -> [w708 w714]
              tunnel: [w708 w714] -> w686
              frame False {
                n241 = call "SetupInterfArrDev.vi"("error in (no error)"=w710, "Experiment.lvclass"=w711, "DevID"=w709, "Interface en entrée"=w712) -> ("error out"=w713:errorcluster, "Interface en sortie"=w707:refnum<class "Interface.lvclass">)  [unwired: 5 in, 1 out]
              }
              frame True {
                n242 = One Button Dialog(message="This device doesn't have array functions ") -> ()  [unwired: 1 in, 1 out]
              }
            }
          }
        }
      }
      n243 = while {
        shift-right: [w26] -> w13
        shift-left: w15 -> [w27]
        tunnel: w19 -> [w28]
        stop <- w24 stop-if-true
        n244 = event shown="[4] \"SaveCurvePar\": Valeur changée" {
          selector: _ -> [_ _ _ _ _ _ _ _ _ _ _ _ _ _ _]
          dyn-events: _ -> [_ _ _ _ _ _ _ _ _ _ _ _ _ _ _]
          timeout: 200 -> [_ _ _ _ _ _ _ _ _ _ _ _ _ _ _]
          tunnel: w28 -> [_ _ _ w72 w77 w89 _ _ _ w189 w217 w233 w236 w249 w252]
          tunnel: w27 -> [w30 w51 w53 w74 w76 w94 w114 w158 w187 w198 w219 w232 w235 w248 w253]
          tunnel: [w30 w49 w52 w73 w75 w90 w111 w153 w187 w190 w218 w221 w234 w246 w250] -> w26
          tunnel: [_ _ _ TRUE _ _ _ _ _ _ _ _ _ _ _] -> w23
          event Timeout {
            n245 = event-data() -> ()  [unwired: 1 in, 2 out]
          }
          event "ParamNaming": Value Change {
            (unwired) "Measurement"
            (unwired) "Instr1."
            w32 = T9."Disabled and Grayed Out" ("Désactivé")
            w34 = T9."Enabled" ("Désactivé")
            n246 = event-data() -> ("NewVal"=w33:bool)  [unwired: 1 in]
            n247 = Select(t=w34, s=w33, f=w32) -> (s? t:f=w31:T9)
            n248 = Select(t=w32, s=w33, f=w34) -> (s? t:f=w35:T9)
            n249 = property on="DisplayName" class="Ch"(error in=w51, "DisabledEnum"=w35) -> (error out=w50:errorcluster)  [unwired: 1 in, 1 out]
            n250 = call "GetScanFormats.vi"("ErrorIn(No Error)"=w50) -> ("sortie d'erreur"=w40:errorcluster, "Cluster"=w48:T3)  [unwired: 8 in, 1 out]
            n251 = Unbundle By Name(w48) -> ("MeasInstrNm"=w36:bool, "MeasUnits"=w38:bool, "ScanSuff"=w42:bool, "ScanParNm"=w43:bool, "2ndScnParNm"=w45:bool, "2ndScnParPos"=w47:bool)
            n252 = property on="2ndVarParPos" class="Bool (strict)"(error in=w40, "Value"=w47, "DisabledEnum"=w31) -> (error out=w46:errorcluster)  [unwired: 1 in, 1 out]
            n253 = property on="2ndScnParNm" class="Bool (strict)"(error in=w46, "Value"=w45, "DisabledEnum"=w31) -> (error out=w44:errorcluster)  [unwired: 1 in, 1 out]
            n254 = property on="ScnInstrNm" class="Bool (strict)"(error in=w44, "Value"=w43, "DisabledEnum"=w31) -> (error out=w41:errorcluster)  [unwired: 1 in, 1 out]
            n255 = property on="ScnLogSffx" class="Bool (strict)"(error in=w41, "Value"=w42, "DisabledEnum"=w31) -> (error out=w39:errorcluster)  [unwired: 1 in, 1 out]
            n256 = property on="MeasUnits" class="Bool (strict)"(error in=w39, "Value"=w38, "DisabledEnum"=w31) -> (error out=w37:errorcluster)  [unwired: 1 in, 1 out]
            n257 = property on="MeasInstrNm" class="Bool (strict)"(error in=w37, "Value"=w36, "DisabledEnum"=w31) -> (error out=w49:errorcluster)  [unwired: 1 in, 1 out]
          }
          event "SaveNamingPar": Value Change {
            n258 = event-data() -> ("NewVal"=w54:bool)  [unwired: 1 in]
            n259 = case shown="Vrai" w54 {
              selector: w54 -> [_ w68]
              tunnel: w53 -> [w55 w66]
              tunnel: [w55 w65] -> w52
              frame False {
              }
              frame True {
                n260 = Not(x=w68) -> (.not. x?=w67:bool)
                n261 = local write "SaveNamingPar"(w67) -> ()
                n262 = Bundle By Name(cluster=T3 {"MeasInstrNm"=FALSE, "MeasUnits"=FALSE, "ScanSuff"=FALSE, "ScanParNm"=FALSE, "2ndScnParNm"=FALSE, "2ndScnParPos"=FALSE} ("Cluster"), "MeasInstrNm"="MeasInstrName", "MeasUnits"="MeasUnits", "ScanSuff"="Scan/Log Suffix", "ScanParNm"="ScanInstrName", "2ndScnParNm"="2ndScanParName", "2ndScnParPos"="2ndVarParPos") -> (w64:T3)
                n263 = call "SetScanFormats.vi"("Cluster"=w64, "Énum"=SetInitPar."ScanFormats", "ErrorIn(No Error)"=w66) -> ("sortie d'erreur"=w65:errorcluster)  [unwired: 12 in]
              }
            }
          }
          event "stop": Value Change; Panel Close {
            n264 = event-data() -> ()  [unwired: 1 in, 2 out]
            n265 = Enqueue Element(queue=w72, element=SetupInterfStates."Stop" ("Énum"), error in (no error)=w74) -> (error out=w73:errorcluster)  [unwired: 1 in, 2 out]
            n266 = local write "stop"(FALSE ("stop")) -> ()
          }
          event "SaveCurvePar": Value Change {
            n267 = event-data() -> ("NewVal"=w78:bool)  [unwired: 1 in, 4 out]
            n268 = case shown="Vrai" w78 {
              selector: w78 -> [_ w88]
              tunnel: w77 -> [_ w86]
              tunnel: w76 -> [w79 w85]
              tunnel: [w79 w80] -> w75
              frame False {
              }
              frame True {
                n269 = Not(x=w88) -> (.not. x?=w87:bool)
                n270 = local write "SaveCurvePar"(w87) -> ()
                n271 = Enqueue Element(queue=w86, element=SetupInterfStates."SaveParams" ("Énum"), error in (no error)=w85) -> (queue out=w81:refnum<queue>, error out=w82:errorcluster)  [unwired: 1 in, 1 out]
                n272 = Enqueue Element(queue=w81, element=SetupInterfStates."2D Graph" ("Énum"), error in (no error)=w82) -> (error out=w80:errorcluster)  [unwired: 1 in, 2 out]
              }
            }
          }
          event "SetGraphConf": Value Change {
            n273 = event-data() -> ("NewVal"=w95:bool)  [unwired: 1 in, 4 out]
            n274 = case shown="Vrai" w95 {
              selector: w95 -> [_ w104]
              tunnel: w94 -> [w96 w102]
              tunnel: [w96 w99] -> w92
              tunnel: w89 -> [_ w97]
              frame False {
              }
              frame True {
                # "must save graph config in class here?"
                n275 = Not(x=w104) -> (.not. x?=w103:bool)
                n276 = local write "SetGraphConf"(w103) -> ()
                n277 = call "SetupGraphConfig.vi"("Error in"=w102) -> ("error out"=w101:errorcluster, "Canceled"=w98:bool, "GraphConfigOut"=w100:i32)  [unwired: 8 in]
                n278 = case shown="Faux" w98 {
                  tunnel: w101 -> [w106 w110]
                  tunnel: w100 -> [w109 _]
                  tunnel: [w105 w110] -> w99
                  tunnel: w97 -> [w108 _]
                  frame False {
                    n279 = local write "Graph Config"(w109) -> ()
                    n280 = Enqueue Element(queue=w108, element=SetupInterfStates."ChngGraphConf" ("Énum"), error in (no error)=w106) -> (error out=w105:errorcluster)  [unwired: 1 in, 2 out]
                  }
                  frame True {
                  }
                }
              }
            }
            n281 = property on="Curve List" class="LstDér (strict)"(error in=w92) -> (error out=w91:errorcluster, "Value"=w93:i32)  [unwired: 1 in, 1 out]
            n282 = property on="Curve List" class="LstDér (strict)"(error in=w91, "Val(Sgnl)"=w93) -> (error out=w90:errorcluster)  [unwired: 1 in, 1 out]
          }
          event "2D Plot": Value Change {
            n283 = event-data() -> ("NewVal"=w115:bool)  [unwired: 1 in, 4 out]
            n284 = control-ref of="2D XScanPar"() -> (w113:refnum<vi>)
            n285 = control-ref of="2D YScanPar"() -> (w112:refnum<vi>)
            n286 = case shown="Faux" w115 {
              tunnel: w114 -> [w127 w143]
              tunnel: w113 -> [w126 w142]
              tunnel: w112 -> [_ w141]
              tunnel: [w120 w133] -> w111
              frame True {
                n287 = Build Array(w126) -> (w129:refnum<vi>[])
                n288 = call <userlib>:"SetCtrlPropGen.vi"("Error in"=w127, "Énum"=T5."Enable", "Controls"=w129) -> ("Error out"=w116:errorcluster)  [unwired: 3 in, 1 out]
                n289 = local read "VarParams"() -> (w125:string[][])
                n290 = call <userlib>:"ArrayTo1DString.vi"("ErrorIn(No Error)"=w116, "DelArrEnd(F)"=TRUE ("DelArrEnd"), "tableau"=w125) -> ("sortie d'erreur"=w117:errorcluster, "Array Out"=w119:string[])  [unwired: 6 in, 1 out]
                n291 = for {
                  tunnel: w119 -> [w132] mode=indexing
                  tunnel: [w131] -> w118 mode=indexing
                  n292 = Match Pattern(string=w132, regular expression="_" ("expression régulière")) -> (before substring=w131:string)  [unwired: 1 in, 3 out]
                }
                n293 = Build Array (concatenate)("Selectionner un Paramètre.." ("PanelIndex"), w118) -> (w122:string[])
                n294 = property on="2D XScanPar" class="MDér (strict)"(error in=w117, "Strings []"=w122) -> (error out=w123:errorcluster)  [unwired: 1 in, 1 out]
                n295 = Merge Errors(w116, w123) -> (w120:errorcluster)
              }
              frame False {
                n296 = Build Array(w142, w141) -> (w135:refnum<vi>[])
                n297 = call <userlib>:"SetCtrlPropGen.vi"("Error in"=w143, "Énum"=T5."DisAndGrayed", "Controls"=w135) -> ("Error out"=w140:errorcluster, "Controls Out"=w139:refnum<vi>[])  [unwired: 3 in]
                n298 = call <userlib>:"SetCtrlPropGen.vi"("Error in"=w140, "Énum"=T6."EnumElementsArr", "Controls"=w139) -> ("Error out"=w137:errorcluster, "Controls Out"=w136:refnum<vi>[])  [unwired: 3 in]
                n299 = call <userlib>:"SetCtrlPropGen.vi"("Error in"=w137, "Énum"=T6."ReinitToDefVal", "Controls"=w136) -> ("Error out"=w133:errorcluster)  [unwired: 3 in, 1 out]
              }
            }
          }
          event "2D XScanPar": Value Change {
            # "xpar line index"
            n300 = event-data() -> ()  [unwired: 1 in, 1 out]
            n301 = control-ref of="2D YScanPar"() -> (w166:refnum<vi>)
            n302 = property on="2D XScanPar" class="MDér (strict)"(error in=w158) -> (error out=w150:errorcluster, "RingText.Text"=w151:string)  [unwired: 1 in, 1 out]
            n303 = local read "VarParams"() -> (w145:string[][])
            n304 = Build Array(w166) -> (w167:refnum<vi>[])
            n305 = call "GetVarParRowCol.vi"("ErrorIn(No Error)"=w150, "VarPar"=w151, "VarParams"=w145) -> ("sortie d'erreur"=w148:errorcluster, "Line"=w147:i32)  [unwired: 6 in, 1 out]
            n306 = property on="2D YScanPar" class="MDér (strict)"(error in=w158) -> (error out=w157:errorcluster, "Value"=w146:u16)  [unwired: 1 in, 1 out]
            n307 = call <userlib>:"SetCtrlPropGen.vi"("Error in"=w150, "Énum"=T5."Enable", "Controls"=w167) -> ("Error out"=w168:errorcluster)  [unwired: 3 in, 1 out]
            n308 = Merge Errors(w148, w168) -> (w149:errorcluster)
            n309 = Equal To 0?(x=w147) -> (x = 0?=→"Fill Line First":bool)
            n310 = Delete From Array(array=w145, index (row)=w147) -> (array with subset deleted=w170:string[][])  [unwired: 2 in, 1 out]
            n311 = Equal To 0?(x=w146) -> (x = 0?=w155:bool)
            n312 = call <userlib>:"ArrayTo1DString.vi"("ErrorIn(No Error)"=w149, "DelArrEnd(F)"=TRUE ("DelArrEnd"), "tableau"=w170) -> ("sortie d'erreur"=w165:errorcluster, "Array Out"=w156:string[])  [unwired: 6 in, 1 out]
            n313 = case shown="Faux" w155 {
              tunnel: w157 -> [w177 w181]
              tunnel: w156 -> [w173 _]
              tunnel: [w178 u16 0] -> w154
              tunnel: [w177 w181] -> w152
              tunnel: w146 -> [w171 _]
              tunnel: w145 -> [w175 _]
              frame False {
                n314 = call <userlib>:"ArrayTo1DString.vi"("DelArrEnd(F)"=TRUE ("DelArrEnd"), "tableau"=w175) -> ("Array Out"=w174:string[])  [unwired: 7 in, 2 out]
                n315 = Index Array(array=w174, index=w171) -> (element=w172:string)
                n316 = Search 1D Array(1D array=w173, element=w172) -> (index of element=w180:i32)  [unwired: 1 in]
                n317 = To Unsigned Word Integer(number=w180) -> (unsigned 16bit integer=w179:u16)
                n318 = Increment(x=w179) -> (x+1=w178:u16)
              }
              frame True {
              }
            }
            n319 = for {
              tunnel: w156 -> [w185] mode=indexing
              tunnel: [w184] -> w160 mode=indexing
              n320 = Match Pattern(string=w185, regular expression="_" ("expression régulière")) -> (before substring=w184:string)  [unwired: 1 in, 3 out]
            }
            n321 = Build Array (concatenate)("Selectionner un Paramètre.." ("PanelIndex"), w160) -> (w163:string[])
            n322 = property on="2D YScanPar" class="MDér (strict)"(error in=w165, "Strings []"=w163, "Value"=w154) -> (error out=w161:errorcluster)  [unwired: 1 in, 1 out]
            n323 = Merge Errors(w152, w161) -> (w153:errorcluster)
          }
          event "2D YScanPar": Value Change {
            n324 = event-data() -> ("NewVal"=w188:u16)  [unwired: 1 in, 4 out]
            n325 = Greater Than 0?(x=w188) -> (x > 0?=w186:bool)
            n326 = local write "2D Plot Act"(w186) -> ()
          }
          event "Graph Window": Value Change {
            n327 = event-data() -> ("NewVal"=w193:i32)  [unwired: 1 in, 4 out]
            n328 = property on="Graph Window" class="MDér (strict)"() -> ("Strings []"=w200:string[])  [unwired: 2 in, 2 out]
            n329 = Index Array(array=w200, index=w193) -> (element=w195:string)
            n330 = Scan From String(format string="Graph %d" ("chaîne de format"), input string=w195, error in=w198) -> (error out=w197:errorcluster, output 1=w196:i32)  [unwired: 2 in, 2 out]
            n331 = case shown="Pas d'erreur" w197 {
              selector: w197 -> [w202 w213]
              tunnel: w196 -> [w203 _]
              tunnel: w195 -> [_ w210]
              tunnel: [w203 w214] -> w194
              tunnel: [w202 w212] -> w191
              frame No Error {
                n332 = local write "Data Only"(FALSE ("Data Only")) -> ()
              }
              frame Error {
                n333 = Match Pattern(string=w210, regular expression="Scan" ("expression régulière")) -> (offset past match=w208:i32)  [unwired: 1 in, 3 out]
                n334 = Greater Than 0?(x=w208) -> (x > 0?=w207:bool)
                n335 = Equal?(x=w210, y="No Graph") -> (x = y?=w211:bool)
                n336 = Select(t=-3 ("GraphIndex"), s=w207, f=-1 ("GraphIndex")) -> (s? t:f=w204:i32)
                n337 = call <vilib>:"Clear Errors.vi"("error in (no error)"=w213) -> ("error out"=w212:errorcluster)  [unwired: 5 in, 1 out]
                n338 = Select(t=-2 ("GraphIndex"), s=w211, f=w204) -> (s? t:f=w214:i32)
                n339 = local write "Data Only"(w211) -> ()
              }
            }
            n340 = local write "GraphIndex"(w194) -> ()
            n341 = Enqueue Element(queue=w189, element=SetupInterfStates."GetScaleName" ("Énum"), error in (no error)=w191) -> (error out=w190:errorcluster)  [unwired: 1 in, 2 out]
          }
          event "ScanParam": Value Change {
            n342 = event-data() -> ()  [unwired: 1 in, 5 out]
            n343 = Enqueue Element(queue=w217, element=SetupInterfStates."GetScaleName" ("Énum"), error in (no error)=w219) -> (error out=w218:errorcluster)  [unwired: 1 in, 2 out]
          }
          event "Curve List": Value Change {
            n344 = event-data() -> ()  [unwired: 1 in, 5 out]
            n345 = Enqueue Element(queue=w233, element=SetupInterfStates."ReadMeasPar" ("élément"), error in (no error)=w232) -> (queue out=w229:refnum<queue>, error out=w230:errorcluster)  [unwired: 1 in, 1 out]
            n346 = Enqueue Element(queue=w229, element=SetupInterfStates."ReadCurvePar" ("élément"), error in (no error)=w230) -> (queue out=w226:refnum<queue>, error out=w227:errorcluster)  [unwired: 1 in, 1 out]
            n347 = Enqueue Element(queue=w226, element=SetupInterfStates."ReadGraphPar" ("élément"), error in (no error)=w227) -> (queue out=w222:refnum<queue>, error out=w223:errorcluster)  [unwired: 1 in, 1 out]
            n348 = Enqueue Element(queue=w222, element=SetupInterfStates."GetScaleName" ("Énum"), error in (no error)=w223) -> (error out=w221:errorcluster)  [unwired: 1 in, 2 out]
          }
          event "EditArrDev": Value Change {
            n349 = event-data() -> ("NewVal"=w237:bool)  [unwired: 1 in]
            n350 = case shown="Vrai" w237 {
              tunnel: [FALSE ("EditArrDev") FALSE ("EditArrDev")] -> w238
              tunnel: w236 -> [_ w243]
              tunnel: w235 -> [w239 w242]
              tunnel: [w239 w241] -> w234
              frame False {
              }
              frame True {
                n351 = Enqueue Element(queue=w243, element=SetupInterfStates."ArrDevSetup" ("Énum"), error in (no error)=w242) -> (error out=w241:errorcluster)  [unwired: 1 in, 2 out]
              }
            }
            n352 = local write "EditArrDev"(w238) -> ()
          }
          event "XScaleName", "YScaleName": Value Change {
            n353 = event-data() -> ()  [unwired: 1 in, 5 out]
            n354 = Enqueue Element(queue=w249, element=SetupInterfStates."ChgScaleName" ("Énum"), error in (no error)=w248) -> (error out=w246:errorcluster)  [unwired: 1 in, 2 out]
          }
          event "X Scale", "YScale": Value Change {
            n355 = event-data() -> ()  [unwired: 1 in, 5 out]
            n356 = Enqueue Element(queue=w252, element=SetupInterfStates."GetScaleName" ("Énum"), error in (no error)=w253) -> (error out=w250:errorcluster)  [unwired: 1 in, 2 out]
          }
        }
        n357 = Or(x=w23, y="stop") -> (x .or. y?=w24:bool)
      }
      n358 = Merge Errors(w12, w13) -> (w11:errorcluster)
    }
    frame Error {
    }
  }
  "error out" <- w4
  "Interface en sortie" <- w2
